vi "RELAYS Write a  Relay.vi"(6 "ON OFF":bool, 8 "error in (no error)":errorcluster, 9 "Relay IDs":u16, 10 "Dev addr":u8=1 format="%x", 11 "VISA resource name":refnum<visa-resource-name>) -> (0 "error out":errorcluster, 1 "success?":bool, 2 "ack":string, 3 "VISA resource name out":refnum<visa-resource-name>)   [LabVIEW 2016, in "MB _relays.lvlib"]
uses:
  MB _relays.lvlib
  private/gen MB frame_ turn the relay ON_OFF.vi
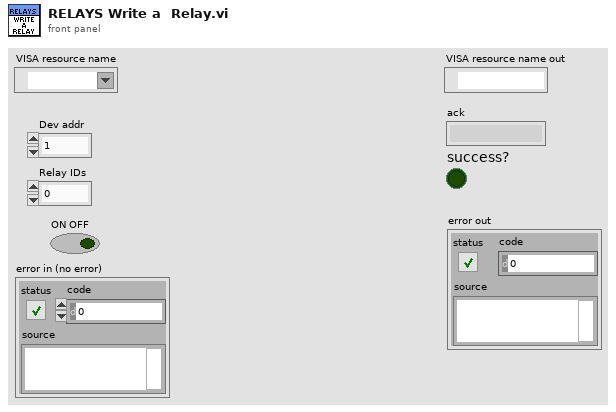
[diagram p1: front panel]
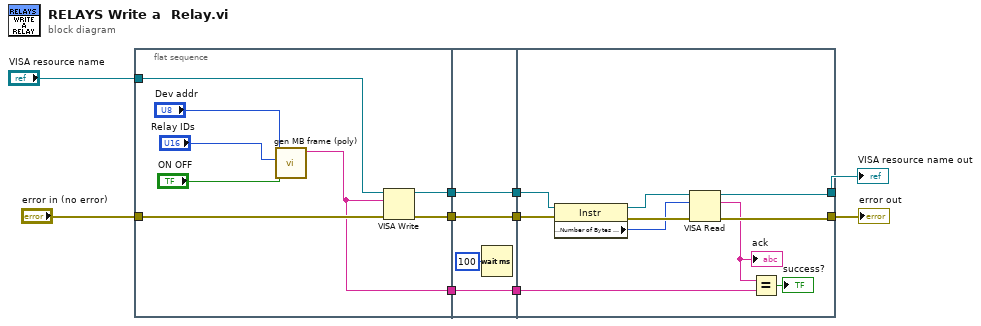
[diagram p0: block diagram]
diagram:
  n1 = flat-sequence {
    tunnel: "error in (no error)" -> [w16]
    tunnel: "VISA resource name" -> [w15]
    tunnel: [w18] -> w6
    tunnel: [w17] -> w5
    tunnel: [w11] -> w1
    tunnel: w6 -> [w22]
    tunnel: w5 -> [w21]
    tunnel: [w22] -> w4
    tunnel: [w21] -> w3
    tunnel: [w19] -> w2
    tunnel: w1 -> [w19]
    tunnel: [w26] -> w9
    tunnel: [w27] -> w10
    tunnel: w4 -> [w31]
    tunnel: w3 -> [w32]
    tunnel: w2 -> [w25]
    frame #0 {
      n2 = call-poly "gen MB frame (poly).vi"("ON OFF"="ON OFF", "Relay IDs"="Relay IDs", "Dev addr"="Dev addr") -> ("MB frame"=w11:string)  [unwired: 8 in]
      n3 = VISA Write(VISA resource name=w15, write buffer=w11, error in (no error)=w16) -> (VISA resource name out=w18:refnum<visa-resource-name>, error out=w17:errorcluster)  [unwired: 1 out]
    }
    frame #1 {
      n4 = Wait (ms)(milliseconds to wait=u32 100) -> ()  [unwired: 1 out]
    }
    frame #2 {
      n5 = property class="Instr"(reference=w31, error in=w32) -> (reference out=w29:refnum<visa-resource-name>, error out=w30:errorcluster, "Serial Settings:Number of Bytes at Serial Port"=w28:u32)
      n6 = VISA Read(VISA resource name=w29, byte count=w28, error in (no error)=w30) -> (VISA resource name out=w27:refnum<visa-resource-name>, read buffer=w24:string, error out=w26:errorcluster)  [unwired: 1 out]
      "ack" <- w24
      n7 = Equal?(x=w24, y=w25) -> (x = y?=→"success?":bool)
    }
  }
  "VISA resource name out" <- w10
  "error out" <- w9
